vi "25-shift_bis_temp.vi"(2 "this":i32, 3 "button":i32) -> (0 "next state":i32, 1 "shift":bool)   [LabVIEW 2017]
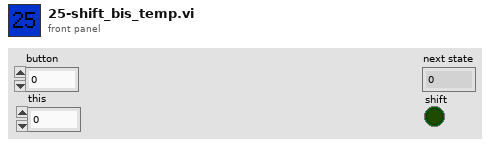
[diagram p1: front panel]
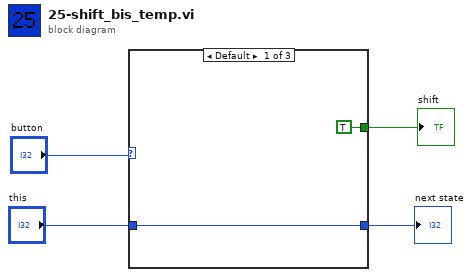
[diagram p0: block diagram]
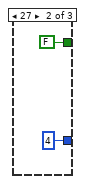
[diagram p2: hidden frame]
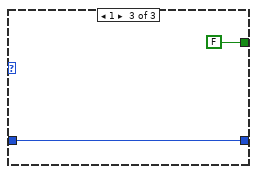
[diagram p3: hidden frame]
diagram:
  n1 = case shown="Default" "button" {
    tunnel: "this" -> [w6 _ w9]
    tunnel: [w6 4 ("this") w9] -> w2
    tunnel: [TRUE FALSE FALSE] -> w1
    frame Default {
    }
    frame 27 {
    }
    frame 1 {
    }
  }
  "next state" <- w2
  "shift" <- w1
